vi "Delete Headers File.vi"(11 "file path (use dialog)":path=path "C:/Snap-On/ModisEdgeScope/Software/Log Results/TEST NAMES LOG.csv") -> (0 "error out":errorcluster)   [LabVIEW 2015]
uses:
  Test Result.ctl
panel:
  in  "Results":T1[](array[typedef])=[{"StepName"="Test Date", "Status"=FALSE, "Data"="", "Limits"=variant}, {"StepName"="Time", "Status"=FALSE, "Data"="", "Limits"=variant}, {"StepName"="SN", "Status"=FALSE, "Data"="", "Limits"=variant}, {"StepName"="Station ID", "Status"=FALSE, "Data"="", "Limits"=variant}, {"StepName"="Fixture ID", "Status"=FALSE, "Data"="", "Limits"=variant}, {"StepName"="Overall Pass/Fail Results", "Status"=FALSE, "Data"="", "Limits"=variant}]
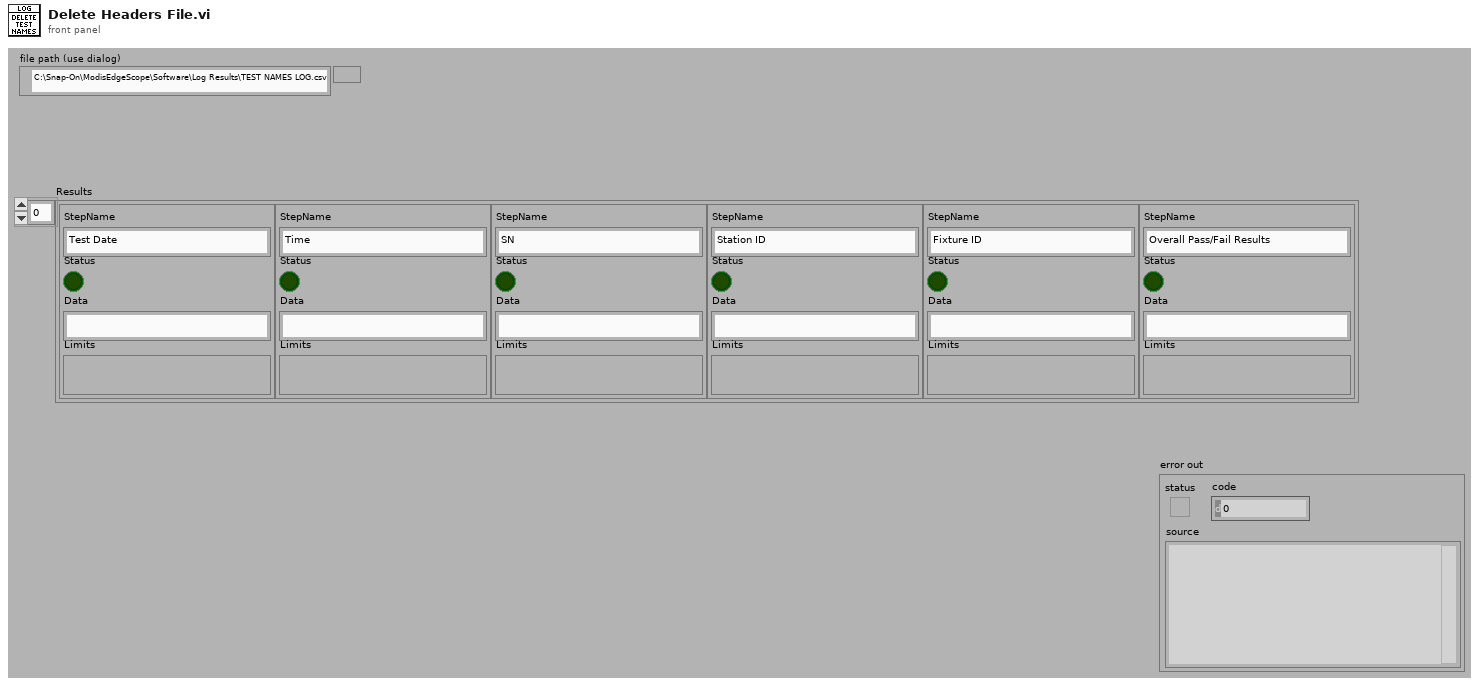
[diagram p1: front panel]
types:
  T1 = typedef "Test Result.ctl" = cluster{"StepName":string, "Status":bool, "Data":string, "Limits":variant}
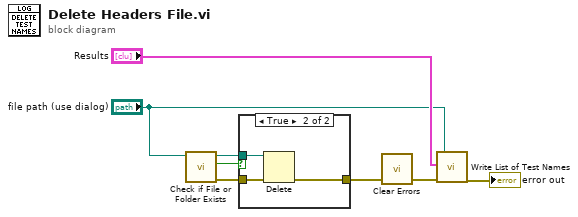
[diagram p0: block diagram]
diagram:
  n1 = call <vilib>:"Check if File or Folder Exists.vi"("path"="file path (use dialog)") -> ("error out"=w4:errorcluster, "file or folder exists?"=w1:bool, "dup path"=w2:path)  [unwired: 8 in]
  n2 = case shown="True" w1 {
    tunnel: [w8 w9] -> w5
    tunnel: w4 -> [w8 w11]
    tunnel: w2 -> [_ w10]
    frame False {
    }
    frame True {
      n3 = Delete(path (use dialog)=w10, error in=w11) -> (error out=w9:errorcluster)  [unwired: 3 in, 2 out]
    }
  }
  n4 = call <vilib>:"Clear Errors.vi"() -> ()  [unwired: 6 in, 2 out]
  n5 = call "Write List of Test Names.vi"("Results"="Results", "error in (no error)"=w5, "file path (use dialog)"="file path (use dialog)") -> ("error out"=→"error out":errorcluster)  [unwired: 16 in]
